vi "RadsRight.vi"(9 "dt":dbl, 10 "Cw2":dbl, 11 "Cw1":dbl) -> (3 "Rs":dbl)   [LabVIEW 2016]
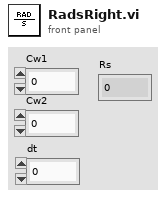
[diagram p1: front panel]
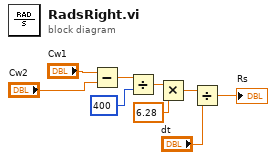
[diagram p0: block diagram]
diagram:
  n1 = Subtract(x="Cw1", y="Cw2") -> (x-y=w9:dbl)
  n2 = Divide(x=w9, y=400) -> (x/y=w7:dbl)
  n3 = Multiply(x=w7, y=6.28) -> (x*y=w5:dbl)
  n4 = Divide(x=w5, y="dt") -> (x/y=→"Rs":dbl)
